vi "PulseHistogram_Relative.vi"(9 "No of SI bins":i32=50, 10 "U8 array probe":u8[](array[numeric]), 11 "Binary array reference":bool[](array[boolean])) -> (3 "Histogram":u64[](array[numeric]))   [LabVIEW 2012]
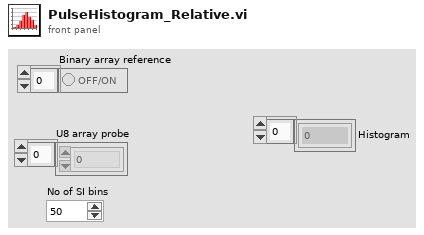
[diagram p1: front panel]
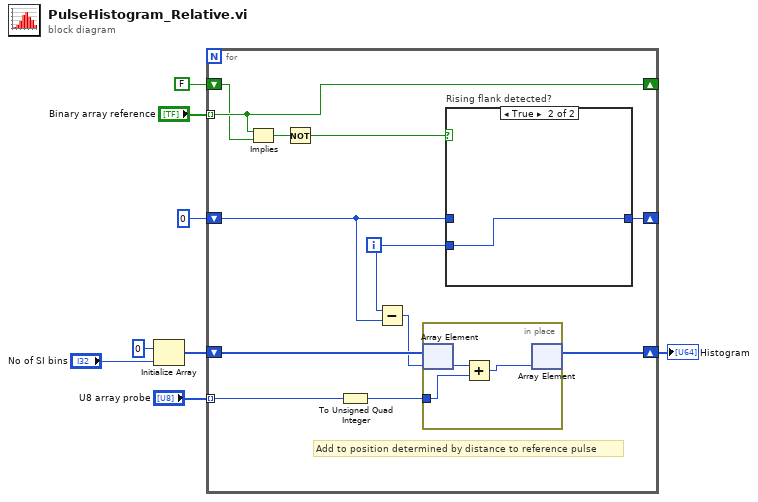
[diagram p0: block diagram]
diagram:
  n1 = Initialize Array(u64 0 ("element"), "No of SI bins") -> (w2:u64[])
  n2 = for {
    tunnel: "Binary array reference" -> [w20] mode=indexing
    shift-right: [w20] -> _
    shift-left: FALSE -> [w19]
    shift-right: [w16] -> _
    shift-left: 0 -> [w14]
    tunnel: "U8 array probe" -> [w11] mode=indexing
    shift-right: [w9] -> w1
    shift-left: w2 -> [w13]
    i -> [w15]
    # "Add to position determined by distance to reference pulse"
    n3 = Implies(1:w19, 2:w20) -> (0:w18:bool)
    n4 = Not(x=w18) -> (.not. x?=w17:bool)
    n5 = To Unsigned Quad Integer(1:w11) -> (0:w10:u64)
    n6 = Subtract(x=w15, y=w14) -> (x-y=w12:i32)
    n7 = in-place {
      in-place-border: w10 -> [w22]
      n8 = in-place-array #1(w13, w12) -> (w23:u64)
      n9 = Add(x=w23, y=w22) -> (x+y=w21:u64)
      n10 = in-place-array #1(w21) -> (w9:u64[])  [unwired: 1 out]
    }
    n11 = case "Rising flank detected?" shown="True" w17 {
      tunnel: w15 -> [_ w25]
      tunnel: [w24 w25] -> w16
      tunnel: w14 -> [w24 _]
      frame False {
      }
      frame True {
      }
    }
  }
  "Histogram" <- w1
